vi "weight_experimental4.vi"(9 "Stop read":bool, 10 "N_points":i32=60, 11 "PV weight":dbl caption="g" format="%#.0f") -> (0 "Weight 3":dbl format="%#.0f", 1 "Q2":dbl format="%#.0f", 2 "Weight 2":dbl format="%#.0f", 3 "Q 1":dbl format="%#.0f", 4 "Q3":dbl format="%#.0f", 5 "Weight 1":dbl format="%#.0f")   [LabVIEW 2019]
uses:
  <vilib>/Analysis/3filter.llb/Filter Passband Type.ctl
  <vilib>/Analysis/baseanly.llb/Mean (DBL).vi
  Logik/fronts.vi
  Trigers/RS.vi
  <vilib>/Analysis/3filter.llb/Butterworth Filter (DBL).vi
  <vilib>/Analysis/NI_AALBase.lvlib
  Timer Delay/Timers.lvlib
panel:
  in  "Tab Control":T1(tab)
  out "dM 2":dbl format="%#.0f"
  out "dM 1":dbl format="%#.0f"
  out "variance":dbl format="%0.2f"
  out "standard deviation":dbl format="%0.2f"
  out "dM 3":dbl format="%#.0f"
  in  "Tare":dbl caption="g" format="%#.0f"
  in  "k":dbl=1.0 caption="g" format="%#.3f"
  # "Усреднение за 1 мин"
  # "(расход)"
  # "Усреднение за 3 мин"
  # "(расход)"
  # "Вес тары\n(полностью очистить бункер от продукта\nи запомнить PV weight или ввести вручную)."
  # "Вес тары\n(ввести фактический вес без учета тары\nили ввести k вручную)"
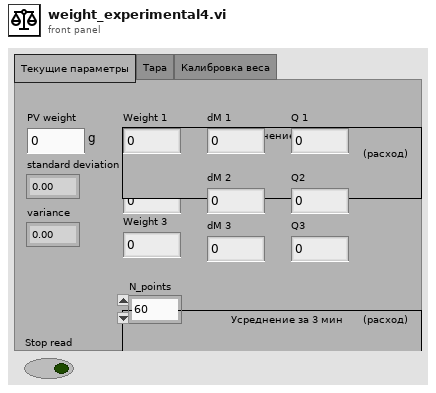
[diagram p1: front panel]
types:
  T1 = enum32{"Текущие параметры", "Тара", "Калибровка веса"}
  T2 = typedef "NI_AALBase.lvlib/Filter Passband Type.ctl" = enum32{"Lowpass", "Highpass", "Bandpass", "Bandstop"}
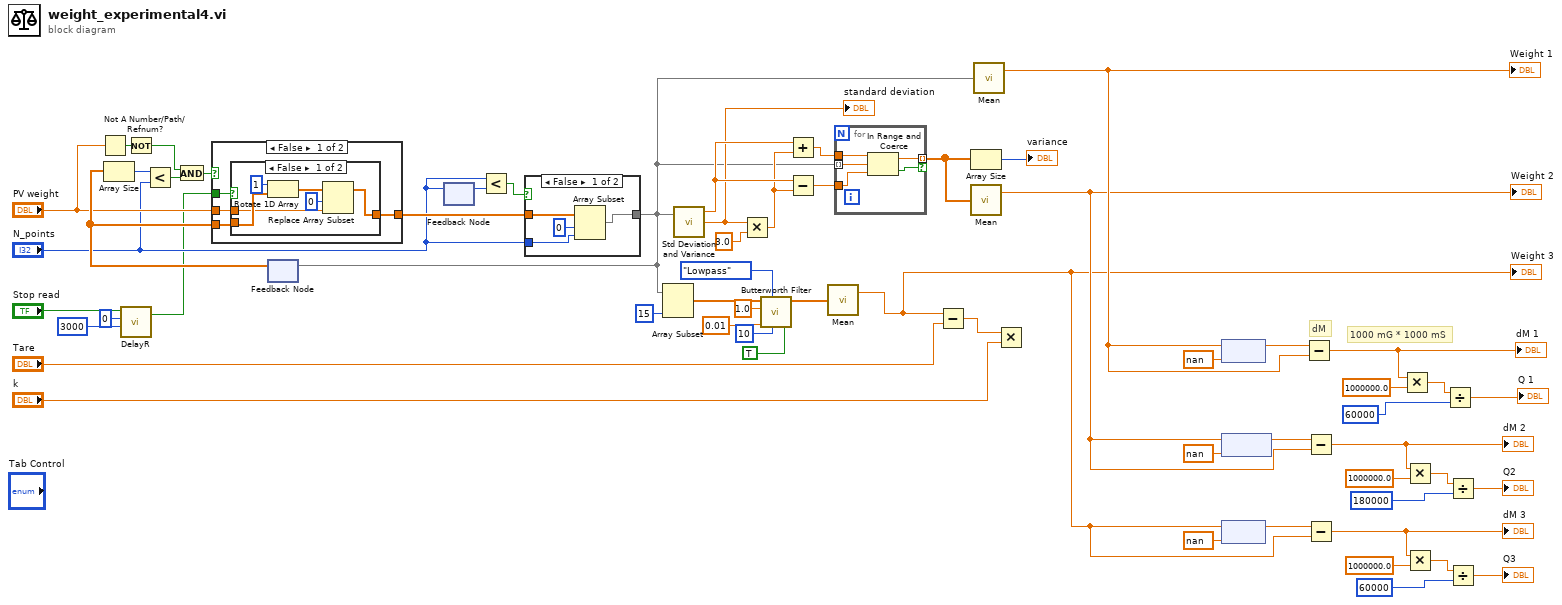
[diagram p0: block diagram]
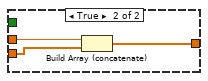
[diagram p4: hidden frame]
diagram:
  # "1000 mG * 1000 mS"
  # "dM"
  n1 = Not A Number/Path/Refnum?(number/path/refnum="PV weight") -> (NaN/Path/Refnum?=w39:bool)
  n2 = call "DelayR.vi"("DelayOff"=u32 3000, "DelayOn"=u32 0, "In"="Stop read") -> ("Out"=w31:bool)  [unwired: 1 in, 1 out]
  n3 = Not(x=w39) -> (.not. x?=w37:bool)
  n4 = feedback #1() -> (w42:dbl[])  [unwired: 1 in]
  n5 = Array Size(array=w42) -> (size(s)=w43:i32)
  n6 = Less?(x=w43, y="N_points") -> (x < y?=w41:bool)
  n7 = And(x=w37, y=w41) -> (x .and. y?=w40:bool)
  n8 = case shown="False" w40 {
    tunnel: [w61 w72] -> w36
    tunnel: "PV weight" -> [w62 w73]
    tunnel: w42 -> [w63 w71]
    tunnel: w31 -> [w60 _]
    frame False {
      n9 = case shown="False" w60 {
        tunnel: w63 -> [w66 w70]
        tunnel: w62 -> [w65 _]
        tunnel: [w64 w70] -> w61
        frame False {
          n10 = Rotate 1D Array(1:w66, 2:1 ("n")) -> (0:w68:dbl[])
          n11 = Replace Array Subset(array=w68, new element=w65, index=0) -> (w64:dbl[])
        }
        frame True {
        }
      }
    }
    frame True {
      n12 = Build Array (concatenate)(w73, w71) -> (w72:dbl[])
    }
  }
  n13 = feedback #2() -> (w34:i32)  [unwired: 1 in]
  n14 = feedback-in #2("N_points") -> ()
  n15 = Less?(x="N_points", y=w34) -> (x < y?=w33:bool)
  n16 = case shown="False" w33 {
    tunnel: [w76 w78] -> w19
    tunnel: w36 -> [w77 w78]
    tunnel: "N_points" -> [w74 _]
    frame False {
      n17 = Array Subset(array=w77, index=0, length=w74) -> (w76:dbl[])
    }
    frame True {
    }
  }
  n18 = feedback-in #1(w19) -> ()
  n19 = Array Subset(array=w19, length=15) -> (w17:dbl[])  [unwired: 1 in]
  n20 = call <vilib>:"Std Deviation and Variance.vi"("X"=w19) -> ("mean"=w50:dbl, "standard deviation"=w46:dbl)  [unwired: 1 in, 1 out]
  "standard deviation" <- w46
  n21 = Multiply(x=w46, y=3.0) -> (x*y=w44:dbl)
  n22 = call-poly <vilib>:"Butterworth Filter.vi"("init/cont (init:F)"=TRUE, "order"=10, "filter type"=Filter_Passband_Type."Lowpass", "low cutoff freq: fl"=0.01, "sampling freq: fs"=1.0, "X"=w17) -> ("Filtered X"=w2:dbl[])  [unwired: 2 in, 1 out]
  n23 = Add(x=w50, y=w44) -> (x+y=w49:dbl)
  n24 = Subtract(x=w50, y=w44) -> (x-y=w48:dbl)
  n25 = call-poly <vilib>:"Mean.vi"("X"=w2) -> ("mean"=w1:dbl)  [unwired: 1 out]
  "Weight 3" <- w1
  n26 = for {
    tunnel: w19 -> [w81] mode=indexing
    tunnel: w49 -> [w83]
    tunnel: w48 -> [w82]
    tunnel: [w80] -> w15 mode=indexing if=w79
    n27 = In Range and Coerce(upper limit=w83, x=w81, lower limit=w82) -> (coerced(x)=w80:dbl, In Range?=w79:bool)
  }
  n28 = Subtract(x=w1, y="Tare") -> (x-y=w16:dbl)
  n29 = Array Size(array=w15) -> (size(s)=→"variance":i32)
  n30 = call-poly <vilib>:"Mean.vi"("X"=w15) -> ("mean"=w10:dbl)  [unwired: 1 out]
  "Weight 2" <- w10
  n31 = call-poly <vilib>:"Mean.vi"("X"=w19) -> ("mean"=w13:dbl)  [unwired: 1 out]
  "Weight 1" <- w13
  n32 = Multiply(x=w16, y="k") -> ()  [unwired: 1 out]
  n33 = feedback #3(nan) -> (w57:dbl)
  n34 = feedback-in #3(w13) -> ()
  n35 = feedback #4(nan) -> (w11:dbl)
  n36 = feedback-in #4(w10) -> ()
  n37 = feedback #5(nan) -> (w9:dbl)
  n38 = feedback-in #5(w1) -> ()
  n39 = Subtract(x=w57, y=w13) -> (x-y=w26:dbl)
  "dM 1" <- w26
  n40 = Subtract(x=w11, y=w10) -> (x-y=w51:dbl)
  "dM 2" <- w51
  n41 = Subtract(x=w9, y=w1) -> (x-y=w5:dbl)
  "dM 3" <- w5
  n42 = Multiply(x=w26, y=1000000.0) -> (x*y=w55:dbl)
  n43 = Multiply(x=w51, y=1000000.0) -> (x*y=w53:dbl)
  n44 = Multiply(x=w5, y=1000000.0) -> (x*y=w3:dbl)
  n45 = Divide(x=w55, y=u32 60000 ("millisecond timer value")) -> (x/y=→"Q 1":dbl)
  n46 = Divide(x=w53, y=u32 180000 ("millisecond timer value")) -> (x/y=→"Q2":dbl)
  n47 = Divide(x=w3, y=u32 60000 ("millisecond timer value")) -> (x/y=→"Q3":dbl)
